vi "4.vi"() -> ()   [LabVIEW 2020]
uses:
  AreaOfHexahedron.ctl
panel:
  out "Hexahedron's area":dbl
  in  "Hexahedron":T1
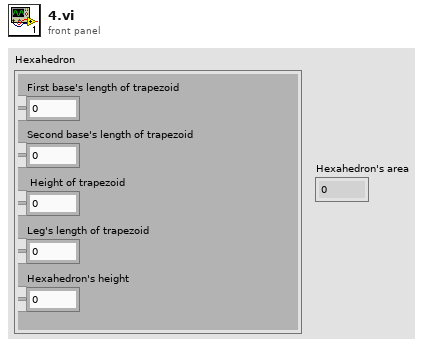
[diagram p1: front panel]
types:
  T1 = typedef "AreaOfHexahedron.ctl" = cluster{"First base's length of trapezoid":dbl, "Second base's length of trapezoid":dbl, " Height of trapezoid":dbl, "Leg's length of trapezoid":dbl, "Hexahedron's height":dbl}
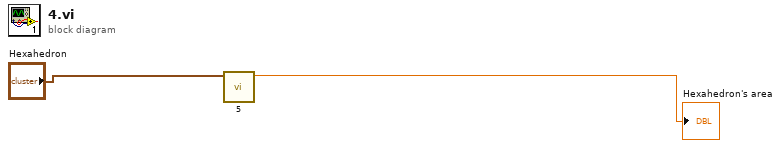
[diagram p0: block diagram]
diagram:
  n1 = call "5.vi"("Hexahedron"="Hexahedron") -> ("Area"=→"Hexahedron's area":dbl)  [unwired: 9 in, 1 out]
